vi "N4_X01_StandartRangeSelect (SubVI).vi"(0 "Range Command":string[](array[string]), 1 "Scale Array":dbl[](array[numeric]), 2 "Range Digit":dbl[](array[numeric]), 3 "Control Point":dbl, 5 "Error In":errorcluster, 6 "RangeAuto":bool=TRUE, 8 "Range":dbl, 9 "Error Code":T2, 11 "Driver Name":T1) -> (14 "Range Out":string, 15 "Scaled value":dbl, 19 "Error Out":errorcluster)   [LabVIEW 2018]
uses:
  MOKO_LabViewLibrary/MokoLowLevel/MokoLowLovelControl/MLLC_ErrorCode.ctl
  MOKO_LabViewLibrary/MokoLowLevel/MokoLowLovelControl/MLLC_DriverName.ctl
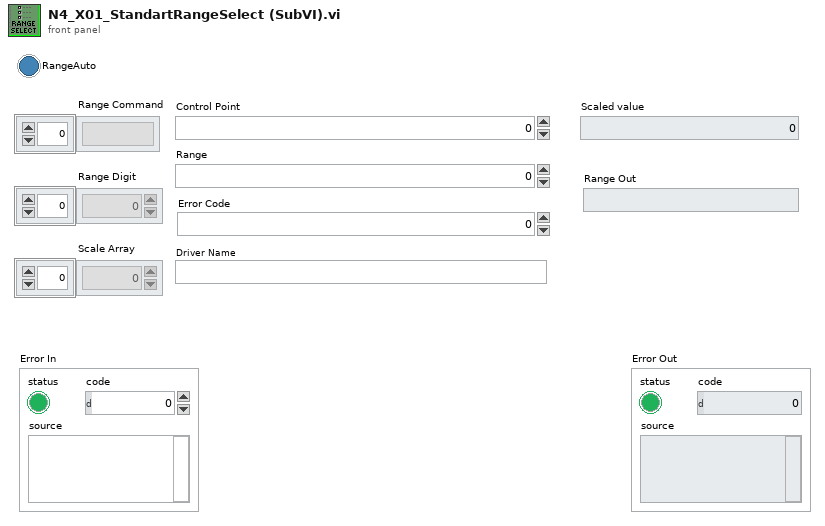
[diagram p1: front panel]
types:
  T1 = typedef "MLLC_DriverName.ctl" = string
  T2 = typedef "MLLC_ErrorCode.ctl" = u32
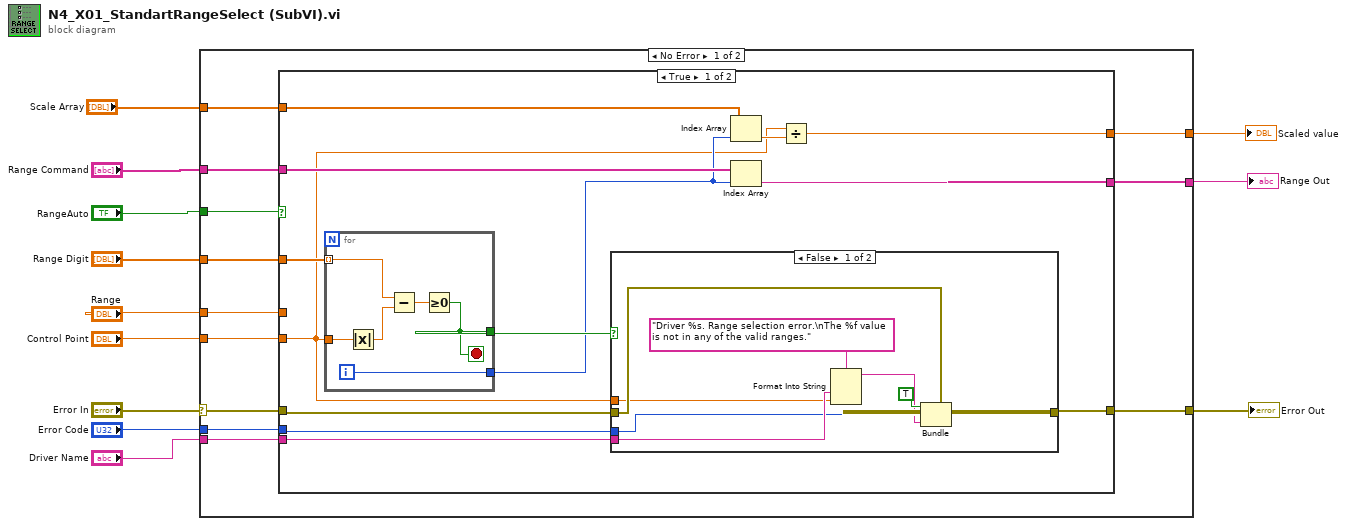
[diagram p0: block diagram]
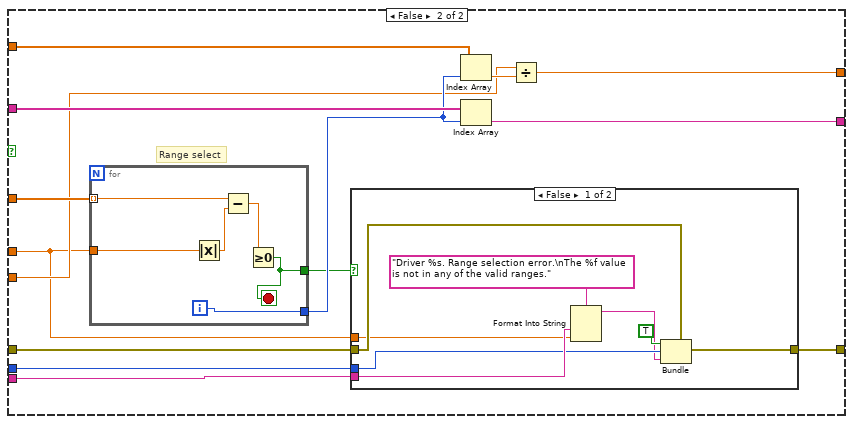
[diagram p3: hidden frame]
diagram:
  n1 = case shown="No Error" "Error In" {
    selector: "Error In" -> [w21 w82]
    tunnel: "Control Point" -> [w16 _]
    tunnel: "Range Digit" -> [w24 _]
    tunnel: "Range Command" -> [w23 _]
    tunnel: [w18 w82] -> w10
    tunnel: [w22 _] -> w2
    tunnel: "Error Code" -> [w19 _]
    tunnel: "Driver Name" -> [w20 _]
    tunnel: "Scale Array" -> [w17 _]
    tunnel: [w15 _] -> w1
    tunnel: "RangeAuto" -> [w14 _]
    tunnel: "Range" -> [w13 _]
    frame No Error {
      n2 = case shown="True" w14 {
        tunnel: w24 -> [w37 w66]
        tunnel: w23 -> [w36 w65]
        tunnel: [w34 w64] -> w22
        tunnel: w21 -> [w33 w57]
        tunnel: w20 -> [w32 w53]
        tunnel: w19 -> [w31 w54]
        tunnel: [w30 w58] -> w18
        tunnel: w17 -> [w29 w63]
        tunnel: w16 -> [w26 w59]
        tunnel: [w25 w60] -> w15
        tunnel: w13 -> [_ w56]
        frame True {
          n3 = for {
            tunnel: w37 -> [w52] mode=indexing
            tunnel: w26 -> [w51]
            tunnel: [w48] -> w28
            tunnel: [w47] -> w35
            i -> [w48]
            stop <- w47 stop-if-true
            n4 = Absolute Value(x=w51) -> (abs(x)=w50:dbl)
            n5 = Subtract(x=w52, y=w50) -> (x-y=w49:dbl)
            n6 = Greater Or Equal To 0?(x=w49) -> (x >= 0?=w47:bool)
          }
          n7 = case shown="False" w35 {
            tunnel: w33 -> [w41 w46]
            tunnel: w32 -> [w43 _]
            tunnel: w31 -> [w40 _]
            tunnel: w26 -> [w39 _]
            tunnel: [w42 w46] -> w30
            frame False {
              n8 = Format Into String(format string="Driver %s. Range selection error.\nThe %f value is not in any of the valid ranges.", w43, w39) -> (resulting string=w38:string)  [unwired: 2 in, 1 out]
              n9 = Bundle(cluster=w41, "status"=TRUE ("Status"), "code"=w40, "source"=w38) -> (w42:errorcluster)
            }
            frame True {
            }
          }
          n10 = Index Array(array=w29, index=w28) -> (element=w27:dbl)
          n11 = Index Array(array=w36, index=w28) -> (element=w34:string)
          n12 = Divide(x=w26, y=w27) -> (x/y=w25:dbl)
        }
        frame False {
          # "Range select"
          n13 = for {
            tunnel: w66 -> [w81] mode=indexing
            tunnel: w56 -> [w80]
            tunnel: [w77] -> w62
            tunnel: [w76] -> w55
            i -> [w77]
            stop <- w76 stop-if-true
            n14 = Absolute Value(x=w80) -> (abs(x)=w79:dbl)
            n15 = Subtract(x=w81, y=w79) -> (x-y=w78:dbl)
            n16 = Greater Or Equal To 0?(x=w78) -> (x >= 0?=w76:bool)
          }
          n17 = case shown="False" w55 {
            tunnel: w57 -> [w70 w75]
            tunnel: w53 -> [w72 _]
            tunnel: w54 -> [w69 _]
            tunnel: w56 -> [w68 _]
            tunnel: [w71 w75] -> w58
            frame False {
              n18 = Format Into String(format string="Driver %s. Range selection error.\nThe %f value is not in any of the valid ranges.", w72, w68) -> (resulting string=w67:string)  [unwired: 2 in, 1 out]
              n19 = Bundle(cluster=w70, "status"=TRUE ("Status"), "code"=w69, "source"=w67) -> (w71:errorcluster)
            }
            frame True {
            }
          }
          n20 = Index Array(array=w63, index=w62) -> (element=w61:dbl)
          n21 = Index Array(array=w65, index=w62) -> (element=w64:string)
          n22 = Divide(x=w59, y=w61) -> (x/y=w60:dbl)
        }
      }
    }
    frame Error {
    }
  }
  "Error Out" <- w10
  "Range Out" <- w2
  "Scaled value" <- w1
